vi "Convert Image Data to Image.vi"(8 "error in (no error)":errorcluster, 11 "Image Data":T1) -> (0 "error out":errorcluster, 3 "Image Out":refnum<k24>)   [LabVIEW 2020, in "MacroAssert.lvlib" / "Win Util.lvlib"]
uses:
  Win Util.lvlib
  <vilib>/wsapi/NI_WebServices.lvlib
  System.Drawing
  <vilib>/picture/picture.llb/imagedata.ctl
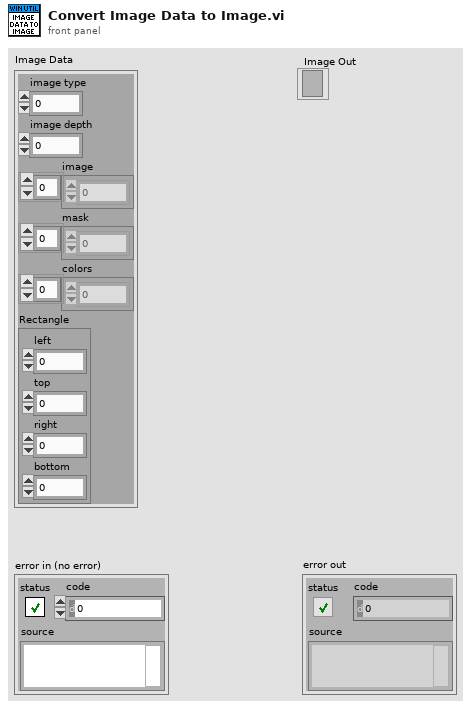
[diagram p1: front panel]
types:
  T1 = typedef "imagedata.ctl" = cluster{"image type":i32, "image depth":i32, "image":u8[], "mask":u8[], "colors":u32[], "Rectangle":cluster{"left":i16, "top":i16, "right":i16, "bottom":i16}}
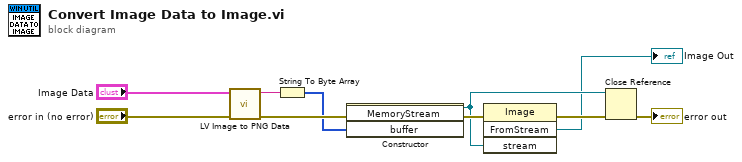
[diagram p0: block diagram]
diagram:
  n1 = call <vilib>:"LV Image to PNG Data.vi"("error in (no error)"="error in (no error)", "image data"="Image Data") -> ("error out"=w5:errorcluster, "png data"=w7:string)  [unwired: 8 in]
  n2 = String To Byte Array(string=w7) -> (unsigned byte array=w4:u8[])
  n3 = constructor class="MemoryStream"(error in=w5, "buffer"=w4) -> (reference out=w3:refnum<k24>, error out=w9:errorcluster)  [unwired: 2 in, 2 out]
  n4 = invoke class="Image" method="FromStream"(error in=w9, "stream"=w3) -> (error out=w8:errorcluster, "FromStream"=→"Image Out":refnum<k24>)  [unwired: 2 in, 2 out]
  n5 = Close Reference(reference=w3, error in (no error)=w8) -> (error out=→"error out":errorcluster)
